vi "Read Part Limits From Configuration.vi"(9 "Test Limits":T1[](array[typedef])=[{"Channel Acquired?"=TRUE, "RMS?"=FALSE, "Pk-Pk"=FALSE, "Frequency"=FALSE, "EU High Limit 1"=0.0, "EU Low Limit 1"=0.0, "EU High Limit 2"=0.0, "EU Low Limit 2"=0.0, "RMS High Limit"=0.0, "RMS Low Limit"=0.0, "Pk-Pk High Limit "=0.0, "Pk-Pk Low Limit"=0.0, "Frequency High Limit"=0.0, "Frequency Low Limit"=0.0}, {"Channel Acquired?"=FALSE, "RMS?"=TRUE, "Pk-Pk"=FALSE, "Frequency"=FALSE, "EU High Limit 1"=0.0, "EU Low Limit 1"=0.0, "EU High Limit 2"=0.0, "EU Low Limit 2"=0.0, "RMS High Limit"=0.0, "RMS Low Limit"=0.0, "Pk-Pk High Limit "=0.0, "Pk-Pk Low Limit"=0.0, "Frequency High Limit"=0.0, "Frequency Low Limit"=0.0}, {"Channel Acquired?"=FALSE, "RMS?"=FALSE, "Pk-Pk"=TRUE, "Frequency"=FALSE, "EU High Limit 1"=0.0, "EU Low Limit 1"=0.0, "EU High Limit 2"=0.0, "EU Low Limit 2"=0.0, "RMS High Limit"=0.0, "RMS Low Limit"=0.0, "Pk-Pk High Limit "=0.0, "Pk-Pk Low Limit"=0.0, "Frequency High Limit"=0.0, "Frequency Low Limit"=0.0}, {"Channel Acquired?"=FALSE, "RMS?"=FALSE, "Pk-Pk"=FALSE, "Frequency"=TRUE, "EU High Limit 1"=0.0, "EU Low Limit 1"=0.0, "EU High Limit 2"=0.0, "EU Low Limit 2"=0.0, "RMS High Limit"=0.0, "RMS Low Limit"=0.0, "Pk-Pk High Limit "=0.0, "Pk-Pk Low Limit"=0.0, "Frequency High Limit"=0.0, "Frequency Low Limit"=0.0}], 11 "All Part Info":T2=[{"Type Name"="", "Type Signal Names"=[], "# Signals"=0, "# Parts"=0, "Part Info"=[]}, {"Type Name"="", "Type Signal Names"=[], "# Signals"=0, "# Parts"=0, "Part Info"=[]}]) -> (3 "Type Test Limits":cluster{T1[]}[](array[cluster]))   [LabVIEW 2019]
uses:
  Type Defs and Controls/Test Limits.ctl
  Type Defs and Controls/All Part Info.ctl
  Type Defs and Controls/Part Info.ctl
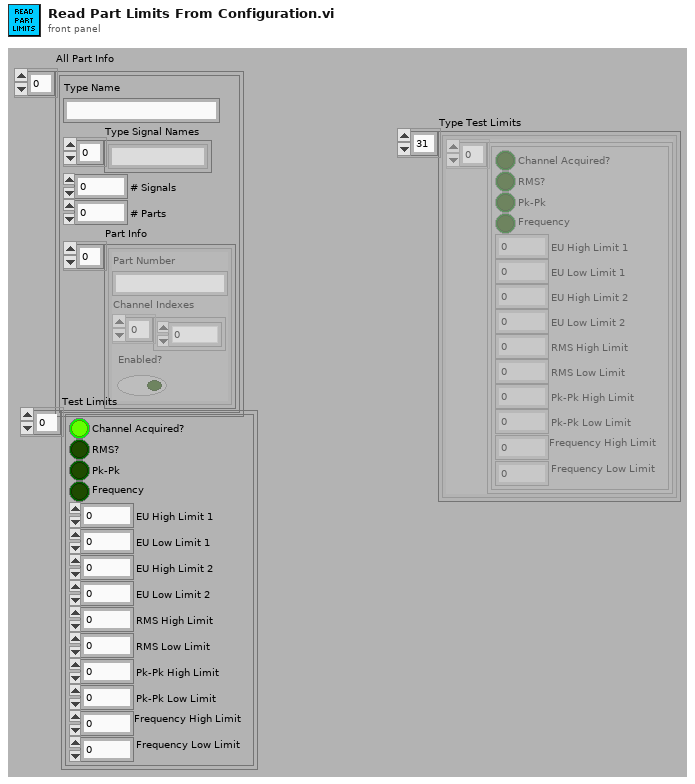
[diagram p1: front panel]
types:
  T1 = typedef "Test Limits.ctl" = cluster{"Channel Acquired?":bool, "RMS?":bool, "Pk-Pk":bool, "Frequency":bool, "EU High Limit 1":dbl, "EU Low Limit 1":dbl, "EU High Limit 2":dbl, "EU Low Limit 2":dbl, "RMS High Limit":dbl, "RMS Low Limit":dbl, "Pk-Pk High Limit ":dbl, "Pk-Pk Low Limit":dbl, "Frequency High Limit":dbl, "Frequency Low Limit":dbl}
  T2 = typedef "All Part Info.ctl" = cluster{"Type Name":string, "Type Signal Names":string[], "# Signals":i32, "# Parts":i32, "Part Info":T3[]}[]
  T3 = typedef "Part Info.ctl" = cluster{"Part Number":string, "Channel Indexes":u16[], "Enabled?":bool}
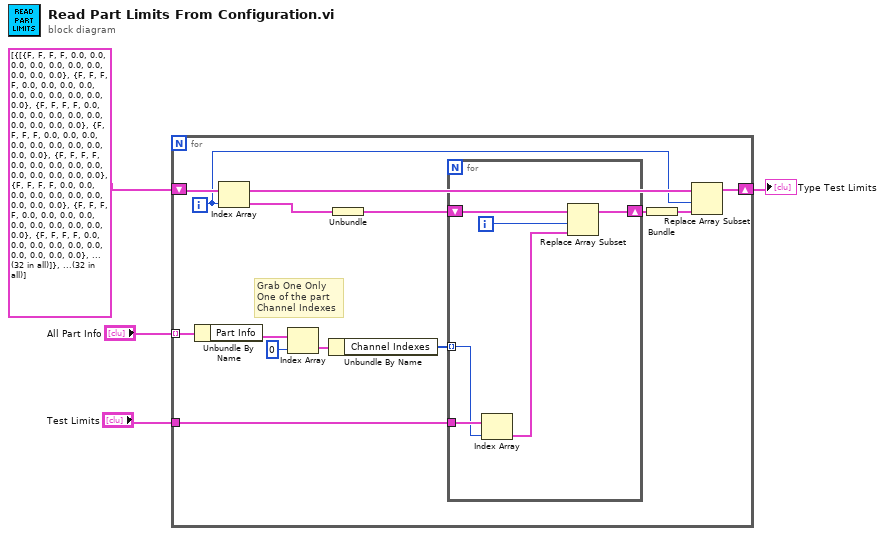
[diagram p0: block diagram]
diagram:
  n1 = for {
    tunnel: "All Part Info" -> [w17] mode=indexing
    tunnel: "Test Limits" -> [w11]
    shift-right: [w5] -> w2
    shift-left: cluster{T1[]}[] [{[{"Channel Acquired?"=FALSE, "RMS?"=FALSE, "Pk-Pk"=FALSE, "Frequency"=FALSE, "EU High Limit 1"=0.0, "EU Low Limit 1"=0.0, "EU High Limit 2"=0.0, "EU Low Limit 2"=0.0, "RMS High Limit"=0.0, "RMS Low Limit"=0.0, "Pk-Pk High Limit "=0.0, "Pk-Pk Low Limit"=0.0, "Frequency High Limit"=0.0, "Frequency Low Limit"=0.0}, {"Channel Acquired?"=FALSE, "RMS?"=FALSE, "Pk-Pk"=FALSE, "Frequency"=FALSE, "EU High Limit 1"=0.0, "EU Low Limit 1"=0.0, "EU High Limit 2"=0.0, "EU Low Limit 2"=0.0, "RMS High Limit"=0.0, "RMS Low Limit"=0.0, "Pk-Pk High Limit "=0.0, "Pk-Pk Low Limit"=0.0, "Frequency High Limit"=0.0, "Frequency Low Limit"=0.0}, {"Channel Acquired?"=FALSE, "RMS?"=FALSE, "Pk-Pk"=FALSE, "Frequency"=FALSE, "EU High Limit 1"=0.0, "EU Low Limit 1"=0.0, "EU High Limit 2"=0.0, "EU Low Limit 2"=0.0, "RMS High Limit"=0.0, "RMS Low Limit"=0.0, "Pk-Pk High Limit "=0.0, "Pk-Pk Low Limit"=0.0, "Frequency High Limit"=0.0, "Frequency Low Limit"=0.0}, {"Channel Acquired?"=FALSE, "RMS?"=FALSE, "Pk-Pk"=FALSE, "Frequency"=FALSE, "EU High Limit 1"=0.0, "EU Low Limit 1"=0.0, "EU High Limit 2"=0.0, "EU Low Limit 2"=0.0, "RMS High Limit"=0.0, "RMS Low Limit"=0.0, "Pk-Pk High Limit "=0.0, "Pk-Pk Low Limit"=0.0, "Frequency High Limit"=0.0, "Frequency Low Limit"=0.0}, {"Channel Acquired?"=FALSE, "RMS?"=FALSE, "Pk-Pk"=FALSE, "Frequency"=FALSE, "EU High Limit 1"=0.0, "EU Low Limit 1"=0.0, "EU High Limit 2"=0.0, "EU Low Limit 2"=0.0, "RMS High Limit"=0.0, "RMS Low Limit"=0.0, "Pk-Pk High Limit "=0.0, "Pk-Pk Low Limit"=0.0, "Frequency High Limit"=0.0, "Frequency Low Limit"=0.0}, {"Channel Acquired?"=FALSE, "RMS?"=FALSE, "Pk-Pk"=FALSE, "Frequency"=FALSE, "EU High Limit 1"=0.0, "EU Low Limit 1"=0.0, "EU High Limit 2"=0.0, "EU Low Limit 2"=0.0, "RMS High Limit"=0.0, "RMS Low Limit"=0.0, "Pk-Pk High Limit "=0.0, "Pk-Pk Low Limit"=0.0, "Frequency High Limit"=0.0, "Frequency Low Limit"=0.0}, {"Channel Acquired?"=FALSE, "RMS?"=FALSE, "Pk-Pk"=FALSE, "Frequency"=FALSE, "EU High Limit 1"=0.0, "EU Low Limit 1"=0.0, "EU High Limit 2"=0.0, "EU Low Limit 2"=0.0, "RMS High Limit"=0.0, "RMS Low Limit"=0.0, "Pk-Pk High Limit "=0.0, "Pk-Pk Low Limit"=0.0, "Frequency High Limit"=0.0, "Frequency Low Limit"=0.0}, {"Channel Acquired?"=FALSE, "RMS?"=FALSE, "Pk-Pk"=FALSE, "Frequency"=FALSE, "EU High Limit 1"=0.0, "EU Low Limit 1"=0.0, "EU High Limit 2"=0.0, "EU Low Limit 2"=0.0, "RMS High Limit"=0.0, "RMS Low Limit"=0.0, "Pk-Pk High Limit "=0.0, "Pk-Pk Low Limit"=0.0, "Frequency High Limit"=0.0, "Frequency Low Limit"=0.0}, {"Channel Acquired?"=FALSE, "RMS?"=FALSE, "Pk-Pk"=FALSE, "Frequency"=FALSE, "EU High Limit 1"=0.0, "EU Low Limit 1"=0.0, "EU High Limit 2"=0.0, "EU Low Limit 2"=0.0, "RMS High Limit"=0.0, "RMS Low Limit"=0.0, "Pk-Pk High Limit "=0.0, "Pk-Pk Low Limit"=0.0, "Frequency High Limit"=0.0, "Frequency Low Limit"=0.0}, {"Channel Acquired?"=FALSE, "RMS?"=FALSE, "Pk-Pk"=FALSE, "Frequency"=FALSE, "EU High Limit 1"=0.0, "EU Low Limit 1"=0.0, "EU High Limit 2"=0.0, "EU Low Limit 2"=0.0, "RMS High Limit"=0.0, "RMS Low Limit"=0.0, "Pk-Pk High Limit "=0.0, "Pk-Pk Low Limit"=0.0, "Frequency High Limit"=0.0, "Frequency Low Limit"=0.0}, {"Channel Acquired?"=FALSE, "RMS?"=FALSE, "Pk-Pk"=FALSE, "Frequency"=FALSE, "EU High Limit 1"=0.0, "EU Low Limit 1"=0.0, "EU High Limit 2"=0.0, "EU Low Limit 2"=0.0, "RMS High Limit"=0.0, "RMS Low Limit"=0.0, "Pk-Pk High Limit "=0.0, "Pk-Pk Low Limit"=0.0, "Frequency High Limit"=0.0, "Frequency Low Limit"=0.0}, {"Channel Acquired?"=FALSE, "RMS?"=FALSE, "Pk-Pk"=FALSE, "Frequency"=FALSE, "EU High Limit 1"=0.0, "EU Low Limit 1"=0.0, "EU High Limit 2"=0.0, "EU Low Limit 2"=0.0, "RMS High Limit"=0.0, "RMS Low Limit"=0.0, "Pk-Pk High Limit "=0.0, "Pk-Pk Low Limit"=0.0, "Frequency High Limit"=0.0, "Frequency Low Limit"=0.0}, {"Channel Acquired?"=FALSE, "RMS?"=FALSE, "Pk-Pk"=FALSE, "Frequency"=FALSE, "EU High Limit 1"=0.0, "EU Low Limit 1"=0.0, "EU High Limit 2"=0.0, "EU Low Limit 2"=0.0, "RMS High Limit"=0.0, "RMS Low Limit"=0.0, "Pk-Pk High Limit "=0.0, "Pk-Pk Low Limit"=0.0, "Frequency High Limit"=0.0, "Frequency Low Limit"=0.0}, {"Channel Acquired?"=FALSE, "RMS?"=FALSE, "Pk-Pk"=FALSE, "Frequency"=FALSE, "EU High Limit 1"=0.0, "EU Low Limit 1"=0.0, "EU High Limit 2"=0.0, "EU Low Limit 2"=0.0, "RMS High Limit"=0.0, "RMS Low Limit"=0.0, "Pk-Pk High Limit "=0.0, "Pk-Pk Low Limit"=0.0, "Frequency High Limit"=0.0, "Frequency Low Limit"=0.0}, {"Channel Acquired?"=FALSE, "RMS?"=FALSE, "Pk-Pk"=FALSE, "Frequency"=FALSE, "EU High Limit 1"=0.0, "EU Low Limit 1"=0.0, "EU High Limit 2"=0.0, "EU Low Limit 2"=0.0, "RMS High Limit"=0.0, "RMS Low Limit"=0.0, "Pk-Pk High Limit "=0.0, "Pk-Pk Low Limit"=0.0, "Frequency High Limit"=0.0, "Frequency Low Limit"=0.0}, {"Channel Acquired?"=FALSE, "RMS?"=FALSE, "Pk-Pk"=FALSE, "Frequency"=FALSE, "EU High Limit 1"=0.0, "EU Low Limit 1"=0.0, "EU High Limit 2"=0.0, "EU Low Limit 2"=0.0, "RMS High Limit"=0.0, "RMS Low Limit"=0.0, "Pk-Pk High Limit "=0.0, "Pk-Pk Low Limit"=0.0, "Frequency High Limit"=0.0, "Frequency Low Limit"=0.0}, {"Channel Acquired?"=FALSE, "RMS?"=FALSE, "Pk-Pk"=FALSE, "Frequency"=FALSE, "EU High Limit 1"=0.0, "EU Low Limit 1"=0.0, "EU High Limit 2"=0.0, "EU Low Limit 2"=0.0, "RMS High Limit"=0.0, "RMS Low Limit"=0.0, "Pk-Pk High Limit "=0.0, "Pk-Pk Low Limit"=0.0, "Frequency High Limit"=0.0, "Frequency Low Limit"=0.0}, {"Channel Acquired?"=FALSE, "RMS?"=FALSE, "Pk-Pk"=FALSE, "Frequency"=FALSE, "EU High Limit 1"=0.0, "EU Low Limit 1"=0.0, "EU High Limit 2"=0.0, "EU Low Limit 2"=0.0, "RMS High Limit"=0.0, "RMS Low Limit"=0.0, "Pk-Pk High Limit "=0.0, "Pk-Pk Low Limit"=0.0, "Frequency High Limit"=0.0, "Frequency Low Limit"=0.0}, {"Channel Acquired?"=FALSE, "RMS?"=FALSE, "Pk-Pk"=FALSE, "Frequency"=FALSE, "EU High Limit 1"=0.0, "EU Low Limit 1"=0.0, "EU High Limit 2"=0.0, "EU Low Limit 2"=0.0, "RMS High Limit"=0.0, "RMS Low Limit"=0.0, "Pk-Pk High Limit "=0.0, "Pk-Pk Low Limit"=0.0, "Frequency High Limit"=0.0, "Frequency Low Limit"=0.0}, {"Channel Acquired?"=FALSE, "RMS?"=FALSE, "Pk-Pk"=FALSE, "Frequency"=FALSE, "EU High Limit 1"=0.0, "EU Low Limit 1"=0.0, "EU High Limit 2"=0.0, "EU Low Limit 2"=0.0, "RMS High Limit"=0.0, "RMS Low Limit"=0.0, "Pk-Pk High Limit "=0.0, "Pk-Pk Low Limit"=0.0, "Frequency High Limit"=0.0, "Frequency Low Limit"=0.0}, {"Channel Acquired?"=FALSE, "RMS?"=FALSE, "Pk-Pk"=FALSE, "Frequency"=FALSE, "EU High Limit 1"=0.0, "EU Low Limit 1"=0.0, "EU High Limit 2"=0.0, "EU Low Limit 2"=0.0, "RMS High Limit"=0.0, "RMS Low Limit"=0.0, "Pk-Pk High Limit "=0.0, "Pk-Pk Low Limit"=0.0, "Frequency High Limit"=0.0, "Frequency Low Limit"=0.0}, {"Channel Acquired?"=FALSE, "RMS?"=FALSE, "Pk-Pk"=FALSE, "Frequency"=FALSE, "EU High Limit 1"=0.0, "EU Low Limit 1"=0.0, "EU High Limit 2"=0.0, "EU Low Limit 2"=0.0, "RMS High Limit"=0.0, "RMS Low Limit"=0.0, "Pk-Pk High Limit "=0.0, "Pk-Pk Low Limit"=0.0, "Frequency High Limit"=0.0, "Frequency Low Limit"=0.0}, {"Channel Acquired?"=FALSE, "RMS?"=FALSE, "Pk-Pk"=FALSE, "Frequency"=FALSE, "EU High Limit 1"=0.0, "EU Low Limit 1"=0.0, "EU High Limit 2"=0.0, "EU Low Limit 2"=0.0, "RMS High Limit"=0.0, "RMS Low Limit"=0.0, "Pk-Pk High Limit "=0.0, "Pk-Pk Low Limit"=0.0, "Frequency High Limit"=0.0, "Frequency Low Limit"=0.0}, {"Channel Acquired?"=FALSE, "RMS?"=FALSE, "Pk-Pk"=FALSE, "Frequency"=FALSE, "EU High Limit 1"=0.0, "EU Low Limit 1"=0.0, "EU High Limit 2"=0.0, "EU Low Limit 2"=0.0, "RMS High Limit"=0.0, "RMS Low Limit"=0.0, "Pk-Pk High Limit "=0.0, "Pk-Pk Low Limit"=0.0, "Frequency High Limit"=0.0, "Frequency Low Limit"=0.0}, {"Channel Acquired?"=FALSE, "RMS?"=FALSE, "Pk-Pk"=FALSE, "Frequency"=FALSE, "EU High Limit 1"=0.0, "EU Low Limit 1"=0.0, "EU High Limit 2"=0.0, "EU Low Limit 2"=0.0, "RMS High Limit"=0.0, "RMS Low Limit"=0.0, "Pk-Pk High Limit "=0.0, "Pk-Pk Low Limit"=0.0, "Frequency High Limit"=0.0, "Frequency Low Limit"=0.0}, {"Channel Acquired?"=FALSE, "RMS?"=FALSE, "Pk-Pk"=FALSE, "Frequency"=FALSE, "EU High Limit 1"=0.0, "EU Low Limit 1"=0.0, "EU High Limit 2"=0.0, "EU Low Limit 2"=0.0, "RMS High Limit"=0.0, "RMS Low Limit"=0.0, "Pk-Pk High Limit "=0.0, "Pk-Pk Low Limit"=0.0, "Frequency High Limit"=0.0, "Frequency Low Limit"=0.0}, {"Channel Acquired?"=FALSE, "RMS?"=FALSE, "Pk-Pk"=FALSE, "Frequency"=FALSE, "EU High Limit 1"=0.0, "EU Low Limit 1"=0.0, "EU High Limit 2"=0.0, "EU Low Limit 2"=0.0, "RMS High Limit"=0.0, "RMS Low Limit"=0.0, "Pk-Pk High Limit "=0.0, "Pk-Pk Low Limit"=0.0, "Frequency High Limit"=0.0, "Frequency Low Limit"=0.0}, {"Channel Acquired?"=FALSE, "RMS?"=FALSE, "Pk-Pk"=FALSE, "Frequency"=FALSE, "EU High Limit 1"=0.0, "EU Low Limit 1"=0.0, "EU High Limit 2"=0.0, "EU Low Limit 2"=0.0, "RMS High Limit"=0.0, "RMS Low Limit"=0.0, "Pk-Pk High Limit "=0.0, "Pk-Pk Low Limit"=0.0, "Frequency High Limit"=0.0, "Frequency Low Limit"=0.0}, {"Channel Acquired?"=FALSE, "RMS?"=FALSE, "Pk-Pk"=FALSE, "Frequency"=FALSE, "EU High Limit 1"=0.0, "EU Low Limit 1"=0.0, "EU High Limit 2"=0.0, "EU Low Limit 2"=0.0, "RMS High Limit"=0.0, "RMS Low Limit"=0.0, "Pk-Pk High Limit "=0.0, "Pk-Pk Low Limit"=0.0, "Frequency High Limit"=0.0, "Frequency Low Limit"=0.0}, {"Channel Acquired?"=FALSE, "RMS?"=FALSE, "Pk-Pk"=FALSE, "Frequency"=FALSE, "EU High Limit 1"=0.0, "EU Low Limit 1"=0.0, "EU High Limit 2"=0.0, "EU Low Limit 2"=0.0, "RMS High Limit"=0.0, "RMS Low Limit"=0.0, "Pk-Pk High Limit "=0.0, "Pk-Pk Low Limit"=0.0, "Frequency High Limit"=0.0, "Frequency Low Limit"=0.0}, {"Channel Acquired?"=FALSE, "RMS?"=FALSE, "Pk-Pk"=FALSE, "Frequency"=FALSE, "EU High Limit 1"=0.0, "EU Low Limit 1"=0.0, "EU High Limit 2"=0.0, "EU Low Limit 2"=0.0, "RMS High Limit"=0.0, "RMS Low Limit"=0.0, "Pk-Pk High Limit "=0.0, "Pk-Pk Low Limit"=0.0, "Frequency High Limit"=0.0, "Frequency Low Limit"=0.0}, {"Channel Acquired?"=FALSE, "RMS?"=FALSE, "Pk-Pk"=FALSE, "Frequency"=FALSE, "EU High Limit 1"=0.0, "EU Low Limit 1"=0.0, "EU High Limit 2"=0.0, "EU Low Limit 2"=0.0, "RMS High Limit"=0.0, "RMS Low Limit"=0.0, "Pk-Pk High Limit "=0.0, "Pk-Pk Low Limit"=0.0, "Frequency High Limit"=0.0, "Frequency Low Limit"=0.0}]}, ...(32 in all)] ("initialized array") -> [w9]
    i -> [w6]
    # "Grab One Only One of the part Channel Indexes"
    n2 = Unbundle By Name(w17) -> ("Part Info"=w16:T3[])
    n3 = Index Array(array=w9, index=w6) -> (element=w13:cluster{T1[]})
    n4 = Index Array(array=w16, index=0) -> (element=w14:T3)
    n5 = Unbundle By Name(w14) -> ("Channel Indexes"=w12:u16[])
    n6 = Unbundle(w13) -> (w10:T1[])
    n7 = for {
      tunnel: w12 -> [w22] mode=indexing
      shift-right: [w18] -> w8
      shift-left: w10 -> [w21]
      tunnel: w11 -> [w23]
      i -> [w20]
      n8 = Index Array(array=w23, index=w22) -> (element=w19:T1)
      n9 = Replace Array Subset(array=w21, new element=w19, index=w20) -> (w18:T1[])
    }
    n10 = Bundle(w8) -> (w7:cluster{T1[]})  [unwired: 1 in]
    n11 = Replace Array Subset(array=w9, new element=w7, index=w6) -> (w5:cluster{T1[]}[])
  }
  "Type Test Limits" <- w2
